vi "SetSpool_WaitForExtTrigger.vi"(10 "path and name":string, 11 "Kinetic Series":i32) -> ()   [LabVIEW 2018]
panel:
  out "error out (no error)":errorcluster
  out "Return from Start Acquisition":u32
  out "Return from SetSpoolProgress":i32=1
  out "Return from SetSpool":i32=1
  in  "error in (no error)":errorcluster
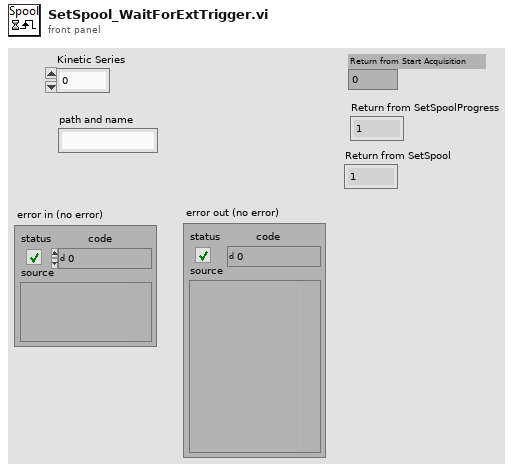
[diagram p1: front panel]
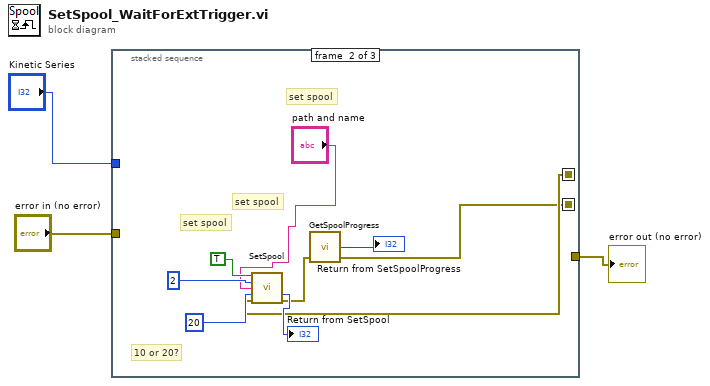
[diagram p0: block diagram]
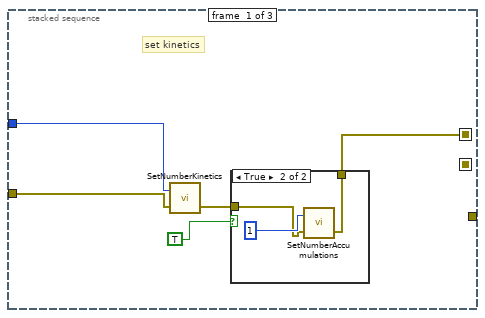
[diagram p2: hidden frame]
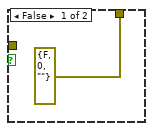
[diagram p3: hidden frame]
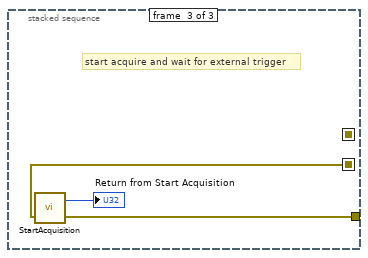
[diagram p4: hidden frame]
diagram:
  n1 = stacked-sequence {
    seq-local: [w4 _ _] -> [_ w15 _]
    seq-local: [_ w14 _] -> [_ _ w23]
    tunnel: "error in (no error)" -> [w8 _ _]
    tunnel: "Kinetic Series" -> [w7 _ _]
    tunnel: [_ _ w22] -> w1
    frame #0 {
      # "set kinetics"
      n2 = call <userlib>:"SetNumberKinetics.vi"("error in (no error)"=w8, "number"=w7) -> ("error out"=w5:errorcluster)  [unwired: 1 out]
      n3 = case shown="True" TRUE {
        tunnel: w5 -> [_ w11]
        tunnel: [errorcluster {"status"=FALSE, "code"=0, "source"=""} ("error in (no error) 2") w10] -> w4
        frame False {
        }
        frame True {
          n4 = call <userlib>:"SetNumberAccumulations.vi"("error in (no error)"=w11, "number"=1) -> ("error out"=w10:errorcluster)  [unwired: 1 out]
        }
      }
    }
    frame #1 {
      # "10 or 20?"
      # "set spool"
      # "set spool"
      # "set spool"
      n5 = call <userlib>:"SetSpool.vi"("active"=TRUE, "method"=2, "name"="path and name", "framebuffersize (10)"=20, "error in (no error)"=w15) -> ("DLL error code"=→"Return from SetSpool":u32, "error out"=w17:errorcluster)  [unwired: 9 in]
      n6 = call <userlib>:"GetSpoolProgress.vi"("error in (no error)"=w17) -> ("error out"=w14:errorcluster, "index"=→"Return from SetSpoolProgress":i32)  [unwired: 2 in, 1 out]
    }
    frame #2 {
      # "start acquire and wait for external trigger"
      n7 = call <userlib>:"StartAcquisition.vi"("error in (no error)"=w23) -> ("error out"=w22:errorcluster, "DLL error code"=→"Return from Start Acquisition":u32)  [unwired: 1 in]
    }
  }
  "error out (no error)" <- w1
